vi "client-test.vi"() -> ()   [LabVIEW 2016]
doc: "cleint test for simple tcp connection. obsolete"
uses:
  <userlib>/_OpenG.lib/error/error.llb/Filter Error Codes (Array)__ogtk.vi
panel:
  out "data out":string
  in  "stop":bool
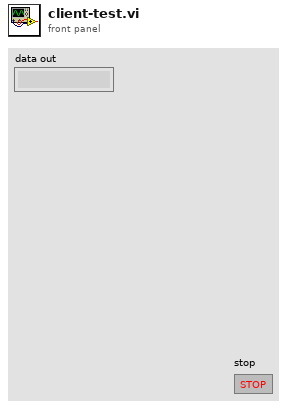
[diagram p1: front panel]
types:
  T1 = enum16{"Standard", "Buffered", "CRLF", "Immediate"}
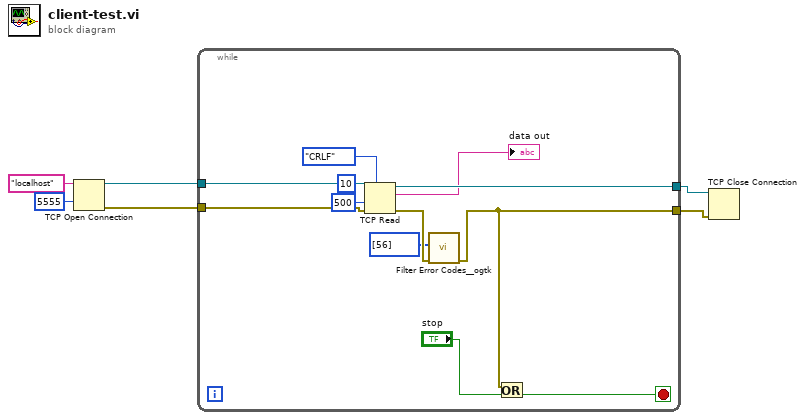
[diagram p0: block diagram]
diagram:
  n1 = TCP Open Connection(address="localhost", remote port or service name=u16 5555) -> (connection ID=w4:refnum<k5>, error out=w2:errorcluster)  [unwired: 3 in]
  n2 = while {
    tunnel: w4 -> [w18]
    tunnel: [w17] -> w3
    tunnel: w2 -> [w16]
    tunnel: [w7] -> w1
    stop <- w8 stop-if-true
    n3 = TCP Read(connection ID=w18, bytes to read=10, error in (no error)=w16, 7:T1."CRLF" ("mode (standard)"), 9:500 ("timeout ms (25000)")) -> (connection ID out=w17:refnum<k5>, data out=→"data out":string, error out=w10:errorcluster)
    n4 = call-poly <userlib>:"Filter Error Codes__ogtk.vi"("Error In"=w10, "Error Codes to Filter"=i32[] [56]) -> ("Error Out"=w7:errorcluster)  [unwired: 7 in, 2 out]
    n5 = Or(x=w7, y="stop") -> (x .or. y?=w8:bool)
  }
  n6 = TCP Close Connection(connection ID=w3, error in (no error)=w1) -> ()  [unwired: 1 in, 2 out]
